vi "Set Perform Action Strategy.vi"(10 "Perform Action Strategy":refnum<class "Perform Action Strategy.lvclass">, 11 "Action Performer in":refnum<class "Virtual Instrument.lvclass">) -> (3 "Action Performer out":refnum<class "Virtual Instrument.lvclass">)   [LabVIEW 2023, in "HAL.lvlib" / "Virtual Instrument.lvclass"]
uses:
  Virtual Instrument.lvclass
  Perform Action Strategy/Perform Action Strategy.lvclass
  Virtual Instrument.lvclass/Virtual Instrument.ctl
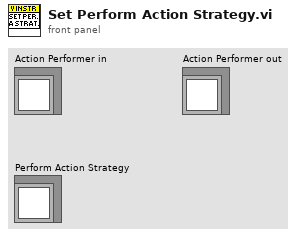
[diagram p1: front panel]
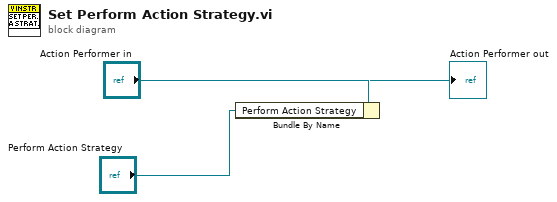
[diagram p0: block diagram]
diagram:
  n1 = Bundle By Name(cluster="Action Performer in", "Perform Action Strategy"="Perform Action Strategy") -> (→"Action Performer out":refnum<class "Virtual Instrument.lvclass">)
